vi "RTS Macro Calc Defrost Time.vi"(7 "Use Filter?":bool=TRUE, 8 "Error In":errorcluster, 9 "Transisition Index":i32, 10 "Input Data":dbl[](array[numeric])) -> (0 "Error Out":errorcluster, 2 "Parsed Output Data":dbl[](array[numeric]), 4 "min value":dbl, 5 "Defrost Time (Min)":dbl, 6 "max value":dbl)   [LabVIEW 2016]
uses:
  <vilib>/gmath/statdist.llb/st_Percentiles (scalar).vi
  <vilib>/gmath/NI_Gmath.lvlib
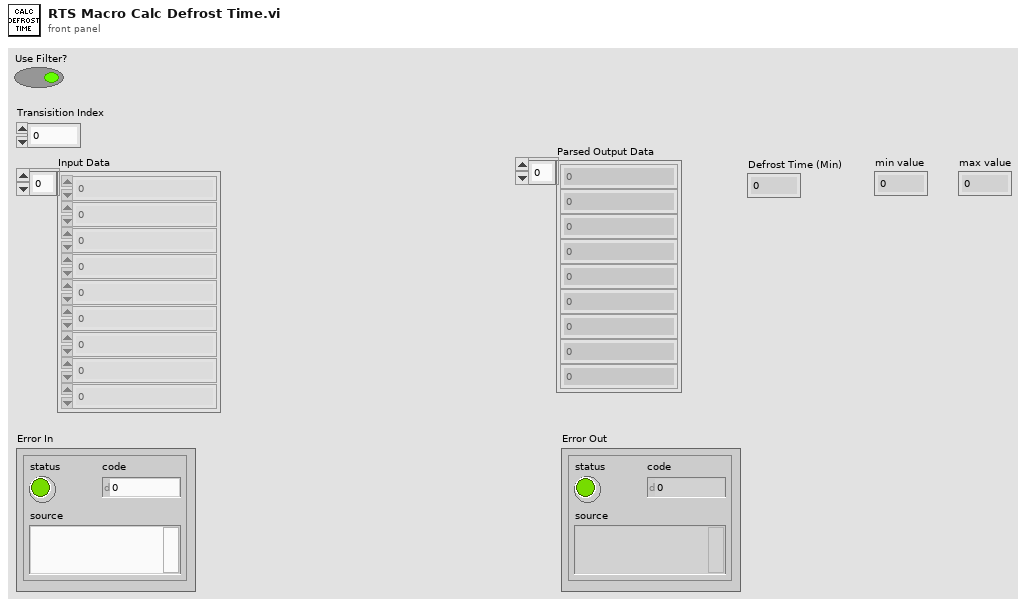
[diagram p1: front panel]
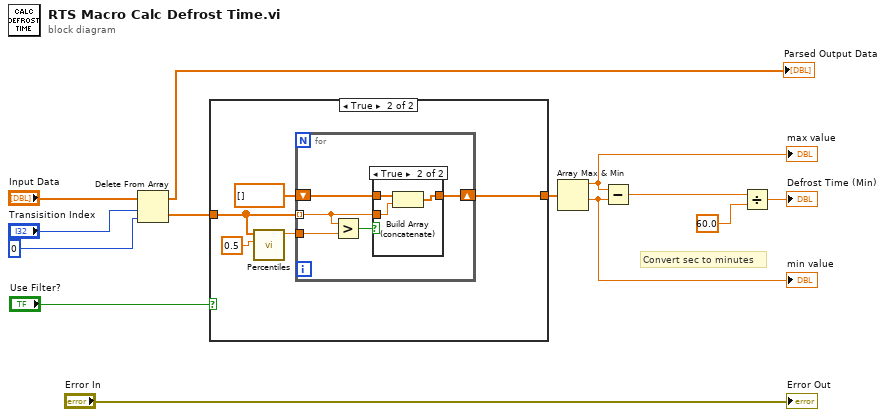
[diagram p0: block diagram]
diagram:
  # "Convert sec to minutes"
  n1 = Delete From Array(array="Input Data", length="Transisition Index", index=0) -> (deleted portion=w3:dbl[], array with subset deleted=→"Parsed Output Data":dbl[])
  n2 = case shown="True" "Use Filter?" {
    tunnel: w3 -> [w14 w18]
    tunnel: [w14 w15] -> w2
    frame False {
    }
    frame True {
      n3 = call-poly <vilib>:"Percentiles.vi"("p"=0.5, "x array"=w18) -> ("percentile"=w17:dbl)  [unwired: 8 in, 1 out]
      n4 = for {
        tunnel: w18 -> [w20] mode=indexing
        tunnel: w17 -> [w24]
        shift-right: [w21] -> w15
        shift-left: dbl[] [] -> [w22]
        n5 = Greater?(x=w20, y=w24) -> (0:w23:bool)
        n6 = case shown="True" w23 {
          tunnel: w22 -> [w25 w28]
          tunnel: [w25 w27] -> w21
          tunnel: w20 -> [_ w26]
          frame False {
          }
          frame True {
            n7 = Build Array (concatenate)(w28, w26) -> (w27:dbl[])
          }
        }
      }
    }
  }
  n8 = Array Max & Min(array=w2) -> (max value=w12:dbl, min value=w13:dbl)  [unwired: 2 out]
  "max value" <- w12
  "min value" <- w13
  n9 = Subtract(x=w12, y=w13) -> (x-y=w5:dbl)
  n10 = Divide(x=w5, y=60.0) -> (x/y=→"Defrost Time (Min)":dbl)
  "Error Out" <- "Error In"
